vi "Connect.vi"(0 "reference in":refnum<class "Database_Postgress.lvclass">, 11 "error in (no error)":errorcluster) -> (4 "reference out":refnum<class "Database_Postgress.lvclass">, 15 "error out":errorcluster)   [LabVIEW 2019, in "Database_Postgress.lvclass"]
uses:
  Database_Postgress.lvclass
  Database_Postgress.lvclass/Database_Postgress.ctl
  Neosoft Technologies/NeoDB for PostgreSQL/Postgres Connector/Postgres Connector.lvclass
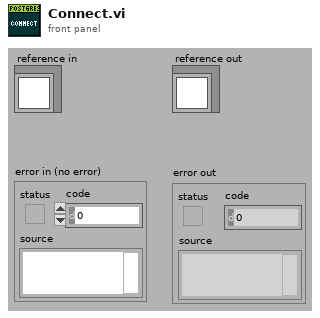
[diagram p1: front panel]
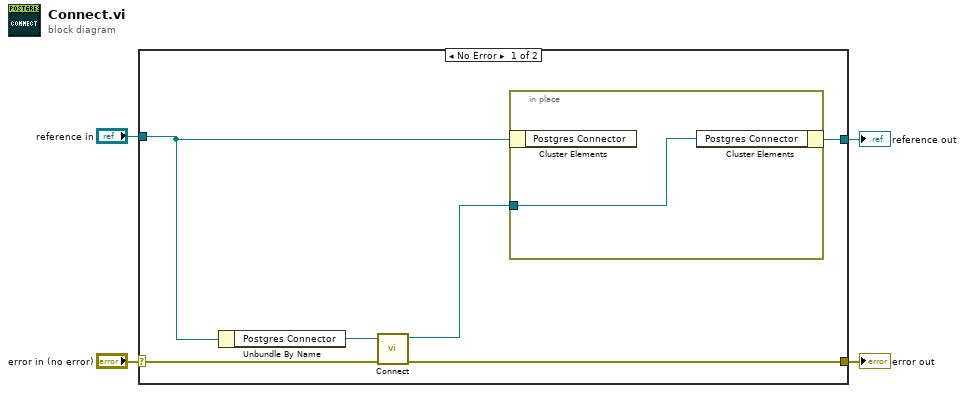
[diagram p0: block diagram]
diagram:
  n1 = case shown="No Error" "error in (no error)" {
    selector: "error in (no error)" -> [w10 w13]
    tunnel: [w7 w13] -> w3
    tunnel: [w5 w12] -> w1
    tunnel: "reference in" -> [w6 w12]
    frame No Error {
      n2 = Unbundle By Name(w6) -> ("Postgres Connector"=w9:refnum<class "Postgres Connector.lvclass">)
      n3 = call "Connect.vi"("error in (no error)"=w10, "Postgres Connector In"=w9) -> ("error out"=w7:errorcluster, "Postgres Connector Out"=w8:refnum<class "Postgres Connector.lvclass">)  [unwired: 8 in]
      n4 = in-place {
        in-place-border: w8 -> [w11]
        n5 = in-place-cluster #1(w6) -> ()  [unwired: 1 out]
        n6 = in-place-cluster #1("Postgres Connector"=w11) -> (w5:refnum<class "Database_Postgress.lvclass">)
      }
    }
    frame Error {
    }
  }
  "error out" <- w3
  "reference out" <- w1
